vi "Table Items to Cluster Array Variant.vi"(0 "Table Items":string[][](array[string]), 2 "Type of Anything":variant, 7 "Columns":T1[](array[typedef]), 11 "error in (no error)":errorcluster) -> (4 "Anything":variant, 15 "error out":errorcluster)   [LabVIEW 2020]
uses:
  ColumnSpec.ctl
  ColumnType.ctl
  Array Manipulation VIs/Array-Dimensions (2D string).vi
  <vilib>/Utility/Data Type/NI_Data Type.lvlib
  KTable.xctl
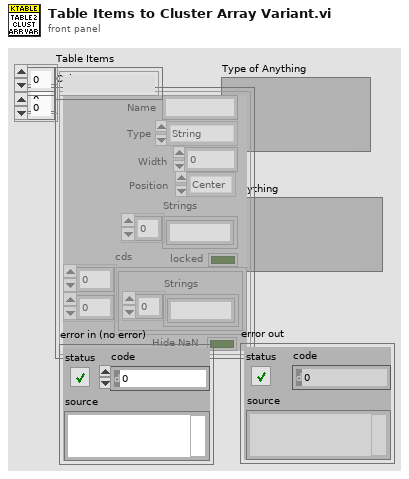
[diagram p1: front panel]
types:
  T1 = typedef "KTable.xctl/ColumnSpec.ctl" = cluster{"Name":string, "Type":T2, "Width":i32, "Strings":string[], "Position":enum16{"Left", "Center", "Right"}, "locked":bool, "cds":cluster{"Strings":string[]}[][], "Hide NaN":bool}
  T2 = typedef "KTable.xctl/ColumnType.ctl" = enum16{"String", "Enum", "Int", "Double", "Boolean", "Ring", "Formula", "Color"}
  T3 = typedef "NI_Data Type.lvlib/Data Type.ctl" = enum8{"Invalid Type", "Void", "I8", "I16", "I32", "I64", "U8", "U16", "U32", "U64", "Single Float", "Double Float", "Extended Float", "Single Complex", "Double Complex", "Extended Complex", "Enum U8", "Enum U16", "Enum U32", "Enum U64", "Single Float With Unit", "Double Float With Unit", "Extended Float With Unit", "Single Complex with Unit", "Double Complex with Unit", "Extended Complex with Unit", "Boolean", "String", "Path", "Picture", "Tag", "Array", "Cluster", "Variant", "LV Variant", "Waveform", "Timestamp", "Digital Waveform", "Digital Data", "ExpressData", "Refnum", "External Data", "VI", "Poly VI", "LabVIEW Class Instance", "Fixed Point", "Set Collection", "Map Collection"}
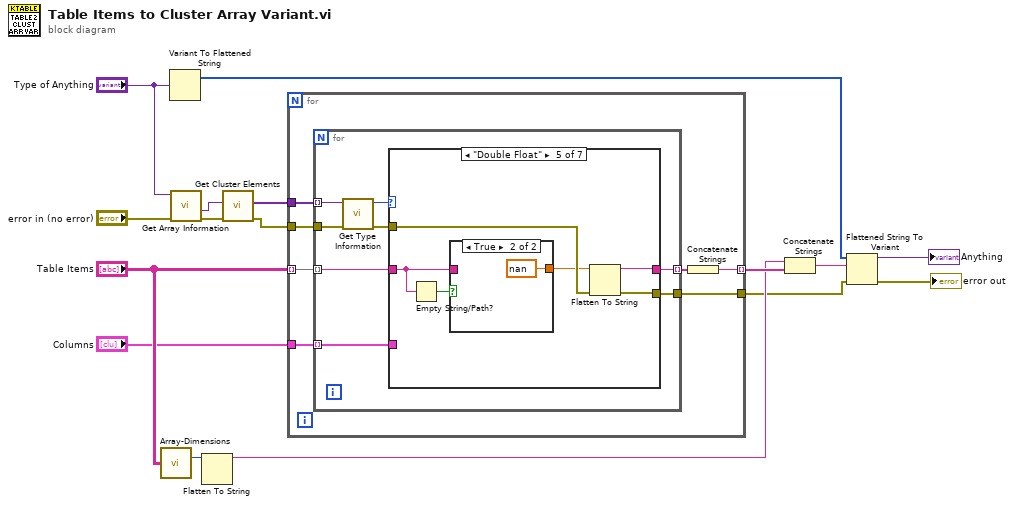
[diagram p0: block diagram]
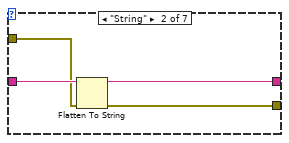
[diagram p3: hidden frame]
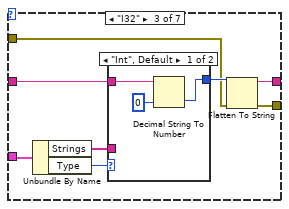
[diagram p4: hidden frame]
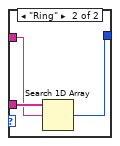
[diagram p5: hidden frame]
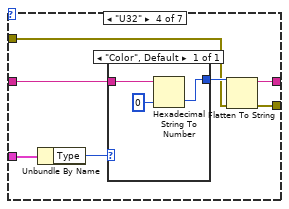
[diagram p6: hidden frame]
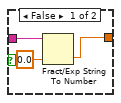
[diagram p7: hidden frame]
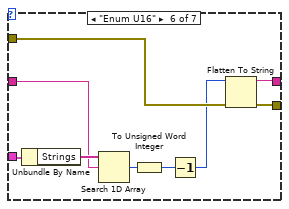
[diagram p8: hidden frame]
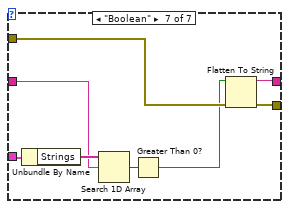
[diagram p9: hidden frame]
diagram:
  n1 = call-poly "Array-Dimensions.vi"("2D Array"="Table Items") -> ("# rows"=w15:i32)  [unwired: 13 in, 1 out]
  n2 = Variant To Flattened String(Variant="Type of Anything") -> (1:w5:i16[])  [unwired: 1 out]
  n3 = call <vilib>:"Get Array Information.vi"("error in (no error)"="error in (no error)", "variant"="Type of Anything") -> ("error out"=w11:errorcluster, "array element data type"=w1:variant)  [unwired: 6 in, 2 out]
  n4 = Flatten To String(anything=w15) -> (data string=w7:string)  [unwired: 3 in, 2 out]
  n5 = call "Get Cluster Elements.vi"("Error In"=w11, "Cluster"=w1) -> ("Error Out"=w10:errorcluster, "Cluster Elements"=w13:variant[])  [unwired: 8 in]
  n6 = for {
    tunnel: "Table Items" -> [w21] mode=indexing
    tunnel: w13 -> [w23]
    tunnel: w10 -> [w22]
    tunnel: "Columns" -> [w20]
    tunnel: [w17] -> w8 mode=indexing
    tunnel: [w18] -> w3
    n7 = for {
      tunnel: w23 -> [w31] mode=indexing
      tunnel: w22 -> [w30]
      tunnel: w21 -> [w29] mode=indexing
      tunnel: w20 -> [w24] mode=indexing
      tunnel: [w27] -> w19 mode=indexing
      tunnel: [w25] -> w18
      n8 = call <vilib>:"Get Type Information.vi"("error in (no error)"=w30, "variant"=w31) -> ("error out"=w26:errorcluster, "type"=w28:T3)  [unwired: 5 in, 3 out]
      n9 = case shown="\"Double Float\"" w28 {
        tunnel: w29 -> [_ w36 w41 w55 w62 w74 w82]
        tunnel: [_ w35 w40 w54 w66 w79 w87] -> w27
        tunnel: w26 -> [w32 w34 w37 w51 w65 w78 w86]
        tunnel: [w32 w33 w39 w53 w64 w77 w85] -> w25
        tunnel: w24 -> [_ _ w44 w57 _ w76 w84]
        frame "Invalid Type", Default {
        }
        frame "String" {
          n10 = Flatten To String(anything=w36, error in (no error)=w34) -> (data string=w35:string, error out=w33:errorcluster)  [unwired: 2 in, 1 out]
        }
        frame "I32" {
          n11 = Unbundle By Name(w44) -> ("Strings"=w42:string[], "Type"=w43:T2)
          n12 = case shown="\"Int\", Default" w43 {
            tunnel: w42 -> [_ w50]
            tunnel: w41 -> [w46 w49]
            tunnel: [w45 w48] -> w38
            frame "Int", Default {
              n13 = Decimal String To Number(string=w46, default (0L)=0 ("default (0 I32)")) -> (number=w45:i32)  [unwired: 1 in, 1 out]
            }
            frame "Ring" {
              n14 = Search 1D Array(1D array=w50, element=w49) -> (index of element=w48:i32)  [unwired: 1 in]
            }
          }
          n15 = Flatten To String(anything=w38, error in (no error)=w37) -> (data string=w40:string, error out=w39:errorcluster)  [unwired: 2 in, 1 out]
        }
        frame "U32" {
          n16 = Unbundle By Name(w57) -> ("Type"=w56:T2)
          n17 = case shown="\"Color\", Default" w56 {
            tunnel: w55 -> [w59]
            tunnel: [w58] -> w52
            frame "Color", Default {
              n18 = Hexadecimal String To Number(string=w59, default (0uL)=u32 0 ("default (0 I32)")) -> (number=w58:u32)  [unwired: 1 in, 1 out]
            }
          }
          n19 = Flatten To String(anything=w52, error in (no error)=w51) -> (data string=w54:string, error out=w53:errorcluster)  [unwired: 2 in, 1 out]
        }
        frame "Double Float" {
          n20 = Empty String/Path?(string/path=w62) -> (empty?=w61:bool)
          n21 = case shown="True" w61 {
            tunnel: [w68 nan] -> w63
            tunnel: w62 -> [w67 _]
            frame False {
              n22 = Fract/Exp String To Number(string=w67, default (0 dbl)=0.0 ("default (0 DBL)")) -> (number=w68:dbl)  [unwired: 2 in, 1 out]
            }
            frame True {
            }
          }
          n23 = Flatten To String(anything=w63, error in (no error)=w65) -> (data string=w66:string, error out=w64:errorcluster)  [unwired: 2 in, 1 out]
        }
        frame "Enum U16" {
          n24 = Unbundle By Name(w76) -> ("Strings"=w75:string[])
          n25 = Search 1D Array(1D array=w75, element=w74) -> (index of element=w73:i32)  [unwired: 1 in]
          n26 = To Unsigned Word Integer(number=w73) -> (unsigned 16bit integer=w72:u16)
          n27 = Decrement(x=w72) -> (x-1=w71:u16)
          n28 = Flatten To String(anything=w71, error in (no error)=w78) -> (data string=w79:string, error out=w77:errorcluster)  [unwired: 2 in, 1 out]
        }
        frame "Boolean" {
          n29 = Unbundle By Name(w84) -> ("Strings"=w83:string[])
          n30 = Search 1D Array(1D array=w83, element=w82) -> (index of element=w81:i32)  [unwired: 1 in]
          n31 = Greater Than 0?(x=w81) -> (x > 0?=w80:bool)
          n32 = Flatten To String(anything=w80, error in (no error)=w86) -> (data string=w87:string, error out=w85:errorcluster)  [unwired: 2 in, 1 out]
        }
      }
    }
    n33 = Concatenate Strings(w19) -> (w17:string)
  }
  n34 = Concatenate Strings(w7, w8) -> (w6:string)
  n35 = Flattened String To Variant(4:w3, 6:w6, 7:w5) -> (0:→"error out":errorcluster, 3:→"Anything":variant)
